vi "Pre Launch Init.vi"(11 "Power Actor in":refnum<class "Power Actor.lvclass">) -> (0 "error out":errorcluster, 3 "Power Actor out":refnum<class "Power Actor.lvclass">)   [LabVIEW 2014, in "Power Library.lvlib" / "Power Actor.lvclass"]
doc: "(<B>Filename</B>: Actor Framework.lvlib:Actor.lvclass:Pre Launch Init.vi)\n\nDefines behavior that occurs after the Launch Nested Actor method is invoked but before the actor's Actor Core method begins running.\n\nBy default, this method does nothing. A descendant class may override it to define behavior."
uses:
  Power Actor.lvclass
  SuperActor/Ex Nested.lvclass
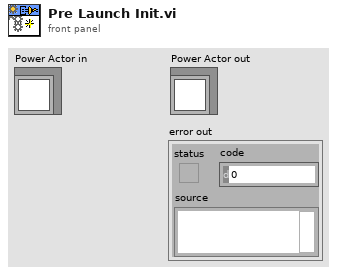
[diagram p1: front panel]
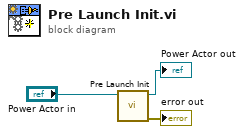
[diagram p0: block diagram]
diagram:
  n1 = call-parent "Pre Launch Init.vi"("Ex Nested in"="Power Actor in") -> ("error out"=→"error out":errorcluster, "Ex Nested out"=→"Power Actor out":refnum<class "Power Actor.lvclass">)  [unwired: 9 in]
